vi "CH_LM Config Wavelength Table Definition.vi"(0 "Meter Index":i32, 2 "Wavelength Table":u32[](array[numeric]), 5 "error in (no error)":errorcluster, 7 "Timeout / ms (3000)":i32=3000, 8 "Action (query)":bool, 9 "Lock Timeout / ms (1000)":i32=1000) -> (11 "Lock timed out":bool, 14 "Meter Index":i32, 16 "Wavelength Table":u32[](array[numeric]), 19 "error out":errorcluster)   [LabVIEW 2012, in "CH_LM.lvlib"]
doc: "This command will set/query the wavelength table entries for the meter. The old list will be replaced by the list of wavelengths specified in the command. Each wavelength will be expressed in units of nm rounded to the nearest integer. Each wavelength will range from 1 to 99999.\n\n<B>Attention:</B> Error 101 will be raised if the list length exceeds 100 entries.\n\n<B>Note</B> that the list returned by the query will always include the calibration wavelength of the current probe."
uses:
  CH_LM.lvlib
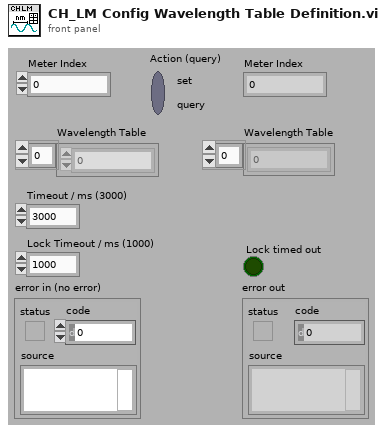
[diagram p1: front panel]
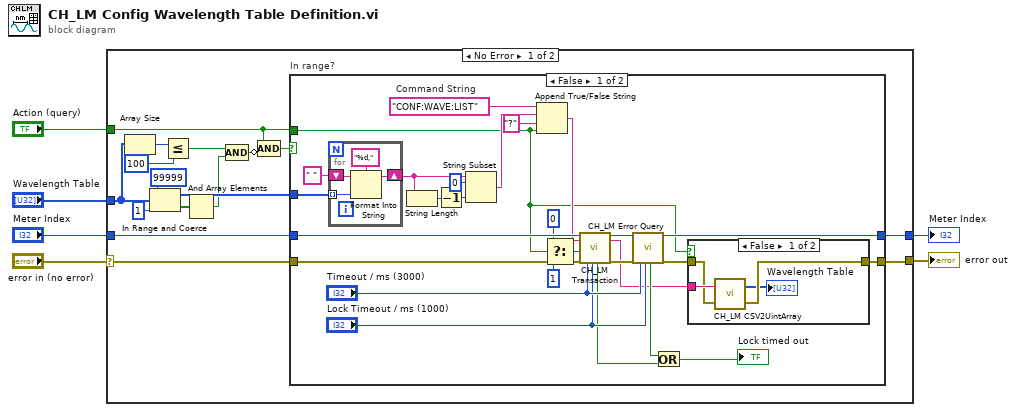
[diagram p0: block diagram]
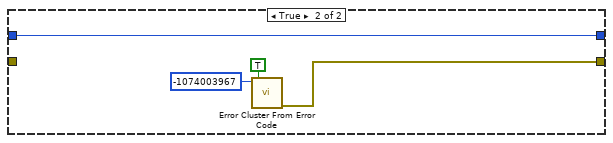
[diagram p3: hidden frame]
diagram:
  n1 = case shown="No Error" "error in (no error)" {
    selector: "error in (no error)" -> [w22 w64]
    tunnel: [w19 w64] -> w6
    tunnel: "Meter Index" -> [w21 w63]
    tunnel: [w20 w63] -> w3
    tunnel: "Action (query)" -> [w10 _]
    tunnel: "Wavelength Table" -> [w16 _]
    frame No Error {
      n2 = Array Size(array=w16) -> (size(s)=w18:i32)
      n3 = In Range and Coerce(upper limit=99999, x=w16, lower limit=1) -> (coerced(x)=w15:u32[], In Range?=w12:bool[])
      n4 = Less Or Equal?(x=w18, y=100) -> (x <= y?=w9:bool)
      n5 = And Array Elements(Boolean array=w12) -> (logical AND=w8:bool)
      n6 = Compound Arithmetic op=AND(w9, w8) -> (w7:bool)
      n7 = Compound Arithmetic op=AND(w10, invert w7) -> (w11:bool)
      n8 = case "In range?" shown="False" w11 {
        tunnel: w22 -> [w49 _]
        tunnel: w21 -> [w48 w62]
        tunnel: [w47 w62] -> w20
        tunnel: w10 -> [w24 _]
        tunnel: w15 -> [w34 _]
        tunnel: [w25 w60] -> w19
        frame False {
          w23 = "CONF:WAVE:LIST"  # Command String
          n9 = for {
            tunnel: w34 -> [w58] mode=indexing
            shift-right: [w56] -> w31
            shift-left: " " ("string (\"\")") -> [w57]
            n10 = Format Into String(format string="%d,", initial string=w57, w58) -> (resulting string=w56:string)  [unwired: 1 in, 1 out]
          }
          n11 = String Length(string=w31) -> (length=w32:i32)
          n12 = Decrement(x=w32) -> (x-1=w30:i32)
          n13 = String Subset(string=w31, offset (0)=0, length (rest)=w30) -> (substring=w28:string)
          n14 = Append True/False String(1:w24, 2:"?", 3:w28, 4:w23) -> (0:w38:string)
          n15 = Select(t=0, s=w24, f=1) -> (s? t:f=w36:i32)
          n16 = call "CH_LM Transaction.vi"("Meter Index"=w48, "Command String"=w38, "NofStrings (-1:all)"=w36, "error in (no error)"=w49, "Timeout / ms (3000)"="Timeout / ms (3000)", "Lock Timeout / ms (1000)"="Lock Timeout / ms (1000)") -> ("Lock timed out"=w41:bool, "Meter Index"=w44:i32, "Response"=w27:string, "error out"=w43:errorcluster)  [unwired: 10 out]
          n17 = call "CH_LM Error Query.vi"("Meter Index"=w44, "error in (no error)"=w43, "Timeout / ms (3000)"="Timeout / ms (3000)", "Lock Timeout / ms (1000)"="Lock Timeout / ms (1000)") -> ("Lock timed out"=w42:bool, "Meter Index"=w47:i32, "error out"=w26:errorcluster)  [unwired: 13 out]
          n18 = Or(x=w42, y=w41) -> (x .or. y?=→"Lock timed out":bool)
          n19 = case shown="False" w24 {
            tunnel: w27 -> [w53 _]
            tunnel: w26 -> [w52 w54]
            tunnel: [w51 w54] -> w25
            frame False {
              n20 = call "CH_LM CSV2UintArray.vi"("error in (no error)"=w52, "CSL"=w53) -> ("error out"=w51:errorcluster, "UInt array"=→"Wavelength Table":u32[])  [unwired: 2 in]
            }
            frame True {
            }
          }
        }
        frame True {
          n21 = call <vilib>:"Error Cluster From Error Code.vi"("show call chain? (False)"=TRUE, "error code (0)"=-1074003967) -> ("error out"=w60:errorcluster)  [unwired: 1 in, 6 out]
        }
      }
    }
    frame Error {
    }
  }
  "error out" <- w6
  "Meter Index" <- w3
